vi "Measure.vi"(8 "error in (no error)":errorcluster, 11 "Temp Monitor in":refnum<class "Standard Measurement.lvclass">) -> (0 "error out":errorcluster, 3 "Temp Monitor out":refnum<class "Standard Measurement.lvclass">)   [LabVIEW 2026, in "Standard Measurement Plugin.lvlib" / "Standard Measurement.lvclass"]
uses:
  Standard Measurement.lvclass
  framework/Measurement Actor/Measurement.lvclass
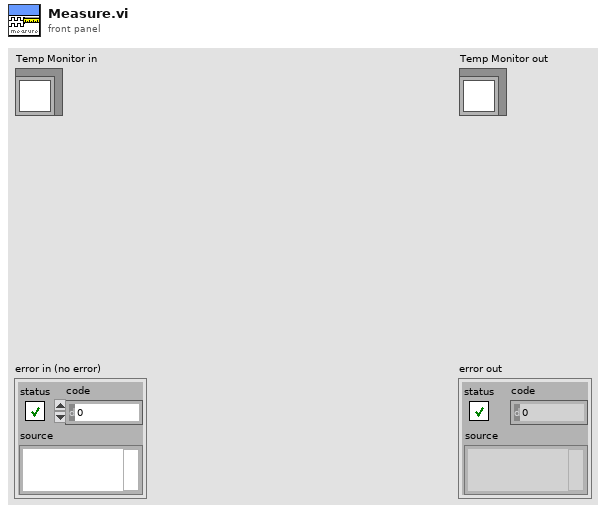
[diagram p1: front panel]
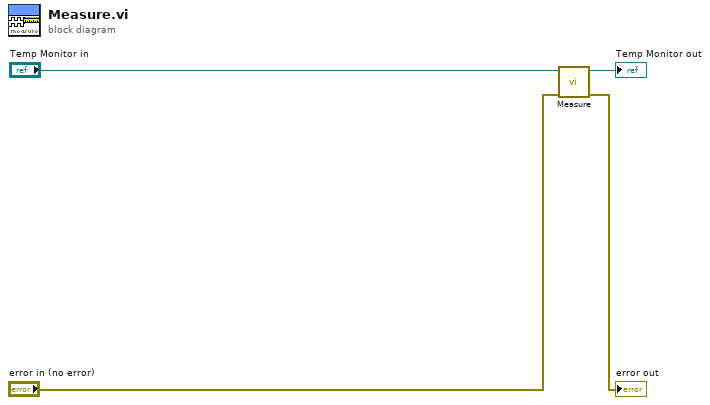
[diagram p0: block diagram]
diagram:
  n1 = call-parent "Measure.vi"("error in (no error)"="error in (no error)", "Measurement in"="Temp Monitor in") -> ("error out"=→"error out":errorcluster, "Measurement out"=→"Temp Monitor out":refnum<class "Standard Measurement.lvclass">)  [unwired: 8 in]
